vi "Close.vi"(8 "error in (no error)":errorcluster, 11 "Kasli Wrapper in":refnum<class "Kasli Wrapper 2.0.lvclass">) -> (0 "error out":errorcluster, 3 "Kasli Wrapper out":refnum<class "Kasli Wrapper 2.0.lvclass">)   [LabVIEW 2020, in "Kasli Wrapper 2.0.lvlib" / "Kasli Wrapper 2.0.lvclass"]
uses:
  Kasli Wrapper 2.0.lvclass
  TALOS/TALOS_PPL.lvlibp
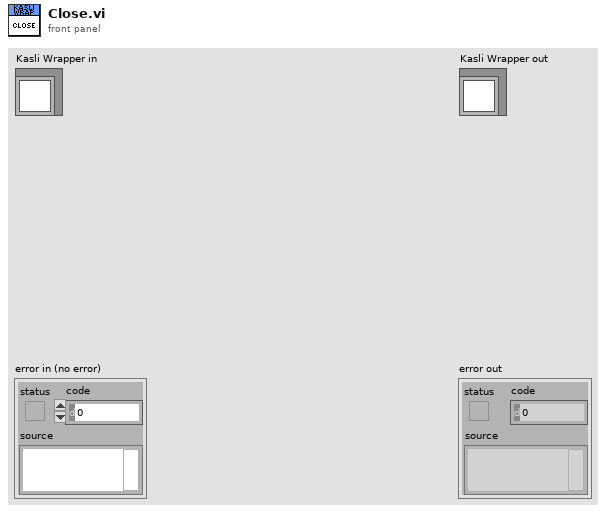
[diagram p1: front panel]
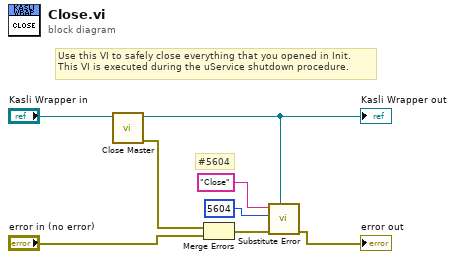
[diagram p0: block diagram]
diagram:
  # "#5604"
  # "Use this VI to safely close everything that you opened in Init.\nThis VI is executed during the uService shutdown procedure."
  n1 = call "Close Master.vi"("Kasli Wrapper 2 in"="Kasli Wrapper in") -> ("error out"=w6:errorcluster, "Kasli Wrapper 2 out"=w1:refnum<class "Kasli Wrapper 2.0.lvclass">)  [unwired: 9 in]
  "Kasli Wrapper out" <- w1
  n2 = Merge Errors(w6, "error in (no error)") -> (w3:errorcluster)
  n3 = call "Substitute Error.vi"("LabVIEW Object"=w1, "error in (no error)"=w3, "Error Code"=5604, "Optional String"="Close") -> ("error out"=→"error out":errorcluster)  [unwired: 7 in]
